vi "Append Page.vi"(6 "Float32 Image":sgl[][](array[numeric]), 7 "U16 Image":u16[][](array[numeric]), 8 "error in (no error)":errorcluster, 9 "I16 Image":i16[][](array[numeric]), 10 "U8 Image":u8[][](array[numeric]), 11 "TIFF File Ref":i32) -> (0 "error out":errorcluster, 3 "TIFF File Ref out":i32)   [LabVIEW 2012]
uses:
  <userlib>/_OpenG.lib/array/array.llb/Empty 2D Array (SGL)__ogtk.vi
  <userlib>/_OpenG.lib/array/array.llb/Empty 2D Array (U16)__ogtk.vi
  <userlib>/_OpenG.lib/array/array.llb/Empty 2D Array (I16)__ogtk.vi
  <userlib>/_OpenG.lib/array/array.llb/Empty 2D Array (U8)__ogtk.vi
  VisualCPP/LabTIFF/Release/LabTIFF.dll
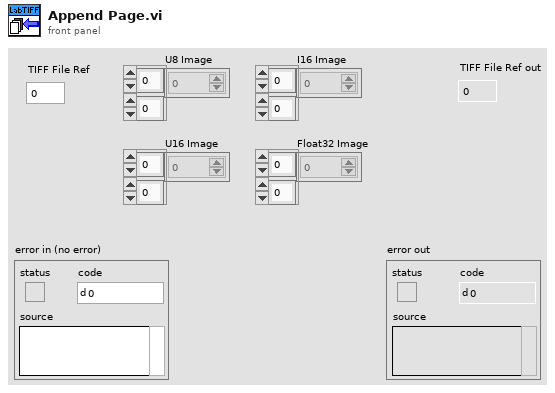
[diagram p1: front panel]
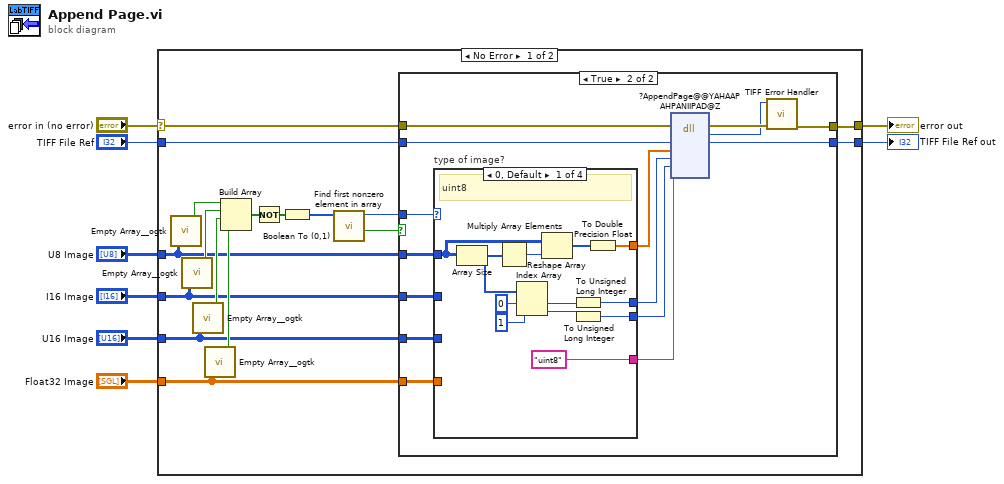
[diagram p0: block diagram]
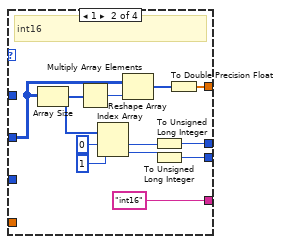
[diagram p3: hidden frame]
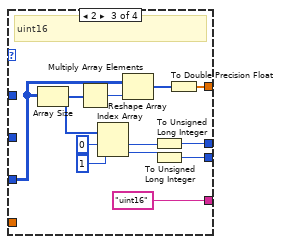
[diagram p4: hidden frame]
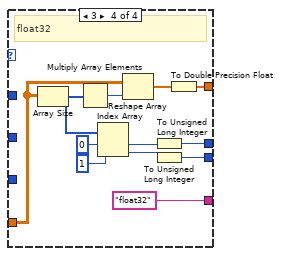
[diagram p5: hidden frame]
diagram:
  n1 = case shown="No Error" "error in (no error)" {
    selector: "error in (no error)" -> [w25 w92]
    tunnel: [w22 w92] -> w7
    tunnel: "TIFF File Ref" -> [w24 w91]
    tunnel: [w23 w91] -> w5
    tunnel: "U8 Image" -> [w12 _]
    tunnel: "I16 Image" -> [w11 _]
    tunnel: "U16 Image" -> [w10 _]
    tunnel: "Float32 Image" -> [w9 _]
    frame No Error {
      n2 = call-poly <userlib>:"Empty Array__ogtk.vi"("Array"=w12) -> ("Empty Array?"=w19:bool)  [unwired: 8 in]
      n3 = call-poly <userlib>:"Empty Array__ogtk.vi"("Array"=w11) -> ("Empty Array?"=w18:bool)  [unwired: 8 in]
      n4 = call-poly <userlib>:"Empty Array__ogtk.vi"("Array"=w10) -> ("Empty Array?"=w17:bool)  [unwired: 8 in]
      n5 = call-poly <userlib>:"Empty Array__ogtk.vi"("Array"=w9) -> ("Empty Array?"=w16:bool)  [unwired: 8 in]
      n6 = Build Array(w19, w18, w17, w16) -> (w15:bool[])
      n7 = Not(x=w15) -> (.not. x?=w14:bool[])
      n8 = Boolean To (0,1)(Boolean=w14) -> (0, 1=w13:i16[])
      n9 = call "Find first nonzero element in array.vi"("Array in"=w13) -> ("found?"=w21:bool, "Index"=w20:i32)  [unwired: 7 in, 2 out]
      n10 = case shown="True" w21 {
        tunnel: w25 -> [w27 w42]
        tunnel: w24 -> [w26 w41]
        tunnel: [w26 w40] -> w23
        tunnel: [w27 w38] -> w22
        tunnel: w20 -> [_ w36]
        tunnel: w12 -> [_ w35]
        tunnel: w11 -> [_ w34]
        tunnel: w10 -> [_ w33]
        tunnel: w9 -> [_ w32]
        frame False {
        }
        frame True {
          n11 = case "type of image?" shown="0, Default" w36 {
            tunnel: w35 -> [w52 _ _ _]
            tunnel: w34 -> [_ w58 _ _]
            tunnel: w33 -> [_ _ w67 _]
            tunnel: w32 -> [_ _ _ w79]
            tunnel: [w51 w55 w68 w80] -> w31
            tunnel: [w47 w57 w70 w82] -> w30
            tunnel: [w45 w56 w69 w81] -> w29
            tunnel: ["uint8" "int16" "uint16" "float32"] -> w28
            frame 0, Default {
              # "uint8"
              n12 = Array Size(array=w52) -> (size(s)=w54:i32[])
              n13 = Multiply Array Elements(1:w54) -> (0:w53:i32)
              n14 = Index Array(array=w54, index #1=0 ("index"), index #2=1 ("index")) -> (element #1=w48:i32, element #2=w46:i32)
              n15 = Reshape Array(w52, w53) -> (w43:u8[])
              n16 = To Unsigned Long Integer(number=w48) -> (unsigned 32bit integer=w47:u32)
              n17 = To Unsigned Long Integer(number=w46) -> (unsigned 32bit integer=w45:u32)
              n18 = To Double Precision Float(number=w43) -> (double precision float=w51:dbl[])
            }
            frame 1 {
              # "int16"
              n19 = Array Size(array=w58) -> (size(s)=w60:i32[])
              n20 = Multiply Array Elements(1:w60) -> (0:w61:i32)
              n21 = Index Array(array=w60, index #1=0 ("index"), index #2=1 ("index")) -> (element #1=w65:i32, element #2=w66:i32)
              n22 = Reshape Array(w58, w61) -> (w62:i16[])
              n23 = To Unsigned Long Integer(number=w65) -> (unsigned 32bit integer=w57:u32)
              n24 = To Unsigned Long Integer(number=w66) -> (unsigned 32bit integer=w56:u32)
              n25 = To Double Precision Float(number=w62) -> (double precision float=w55:dbl[])
            }
            frame 2 {
              # "uint16"
              n26 = Array Size(array=w67) -> (size(s)=w72:i32[])
              n27 = Multiply Array Elements(1:w72) -> (0:w73:i32)
              n28 = Index Array(array=w72, index #1=0 ("index"), index #2=1 ("index")) -> (element #1=w77:i32, element #2=w78:i32)
              n29 = Reshape Array(w67, w73) -> (w74:u16[])
              n30 = To Unsigned Long Integer(number=w77) -> (unsigned 32bit integer=w70:u32)
              n31 = To Unsigned Long Integer(number=w78) -> (unsigned 32bit integer=w69:u32)
              n32 = To Double Precision Float(number=w74) -> (double precision float=w68:dbl[])
            }
            frame 3 {
              # "float32"
              n33 = Array Size(array=w79) -> (size(s)=w84:i32[])
              n34 = Multiply Array Elements(1:w84) -> (0:w85:i32)
              n35 = Index Array(array=w84, index #1=0 ("index"), index #2=1 ("index")) -> (element #1=w89:i32, element #2=w90:i32)
              n36 = Reshape Array(w79, w85) -> (w86:sgl[])
              n37 = To Unsigned Long Integer(number=w89) -> (unsigned 32bit integer=w82:u32)
              n38 = To Unsigned Long Integer(number=w90) -> (unsigned 32bit integer=w81:u32)
              n39 = To Double Precision Float(number=w86) -> (double precision float=w80:dbl[])
            }
          }
          n40 = dll-call lib="C:/Users/Ludo/Programming/Tests/TIFFManagement_test/LabTIFF/VisualCPP/LabTIFF/Release/LabTIFF.dll" fn="?AppendPage@@YAHAAPAHPANIIPAD@Z"(error in=w42, "File Reference"=w41, "Data Array"=w31, "Image Height"=w30, "Image Width"=w29, "Image Type"=w28) -> (error out=w39:errorcluster, "Error"=w37:i32, "File Reference"=w40:i32)  [unwired: 6 in, 1 out]
          n41 = call "TIFF Error Handler.vi"("error in (no error)"=w39, "TIFF DLL error"=w37) -> ("error out"=w38:errorcluster)  [unwired: 9 in]
        }
      }
    }
    frame Error {
    }
  }
  "error out" <- w7
  "TIFF File Ref out" <- w5
